vi "Subset_Array_1D.vi"(9 "Subset Array 1D":i8[](array[numeric])=[0, 1, 2, 3, 4], 10 "Length Subset":i32, 11 "Index Subset":i32) -> (2 "SubArray 1D":i8[](array[numeric]))   [LabVIEW 2018]
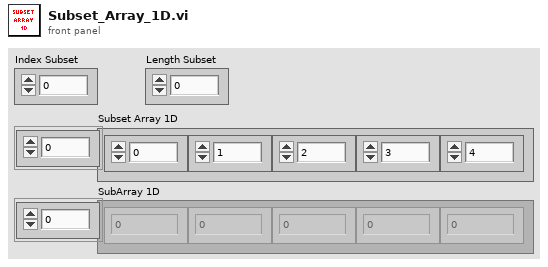
[diagram p1: front panel]
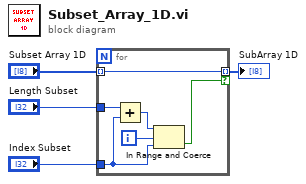
[diagram p0: block diagram]
diagram:
  n1 = for {
    tunnel: "Index Subset" -> [w7]
    tunnel: "Length Subset" -> [w8]
    tunnel: "Subset Array 1D" -> [w6] mode=indexing
    tunnel: [w6] -> w4 mode=indexing if=w5
    i -> [w10]
    n2 = Add(x=w8, y=w7) -> (x+y=w9:i32)
    n3 = In Range and Coerce(upper limit=w9, x=w10, lower limit=w7) -> (In Range?=w5:bool)  [unwired: 1 out]
  }
  "SubArray 1D" <- w4
